vi "Append Section Break to Report.vi"(0 "report in":refnum<class "NI_Standard Report.lvclass">, 11 "error in (no error)":errorcluster) -> (4 "report out":refnum<class "NI_Standard Report.lvclass">, 15 "error out":errorcluster)   [LabVIEW 2020, in "NI_Standard Report.lvclass"]
uses:
  NI_Standard Report.lvclass
  e:/builds/penguin/labview/branches/2020/dev/dist/vi.lib/Utility/NIReport.llb/NI_report.lvclass
  NI_ReportGenerationCore.lvlib
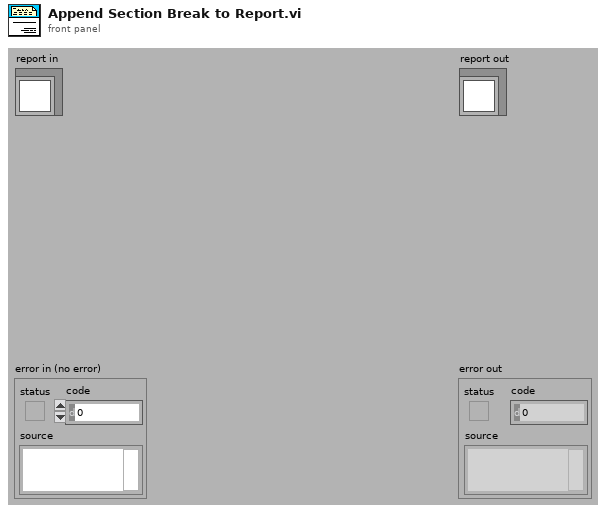
[diagram p1: front panel]
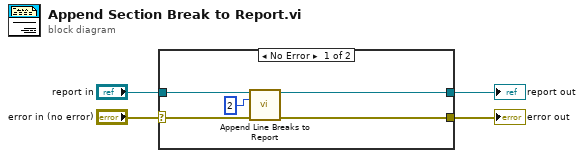
[diagram p0: block diagram]
diagram:
  n1 = case shown="No Error" "error in (no error)" {
    selector: "error in (no error)" -> [w8 w11]
    tunnel: [w5 w11] -> w3
    tunnel: [w6 w10] -> w1
    tunnel: "report in" -> [w9 w10]
    frame No Error {
      n2 = call "Append Line Breaks to Report.vi"("report in"=w9, "number of line breaks"=u32 2 ("Number of line breaks"), "error in (no error)"=w8) -> ("report out"=w6:refnum<class "NI_Standard Report.lvclass">, "error out"=w5:errorcluster)  [unwired: 11 out]
    }
    frame Error {
    }
  }
  "error out" <- w3
  "report out" <- w1
